vi "dlw_Message Log.vi"(6 "Worker Alias":string="Message Log", 7 "Caller in":refnum<class "Worker.lvclass">, 8 "error in":errorcluster, 9 "Initialization Data":T1, 11 "Message Log in":refnum<class "Message Log.lvclass">) -> (0 "error out":errorcluster, 3 "Message Log out":refnum<class "Message Log.lvclass">, 5 "dup Caller out":refnum<class "Worker.lvclass">)   [LabVIEW 2017, in "Message Log.lvclass"]
doc: "This VI dynamically loads the Worker that owns this VI as a subWorker into <b>Caller</b>, and returns the Worker's object containing the Worker's Public Properties. Initialization data that is to be received by this Worker's <Initialize> MHL case can be wired to <b>Initialization Data</b>. The dynamically loaded Worker requires an alias ( <b>Worker Alias</b> ) which must be unique to the Worker it is called from. If a currently loaded subWorker exists with the same Alias, an error will be returned.\n\n<b>Note:</b> This VI can only be called from <b>within</b> another Worker. To call this Worker from an external LabVIEW application, load this Worker with an Asynchronous Launcher VI.\n---"
uses:
  Message Log.lvclass
  C:/Program Files (x86)/National Instruments/LabVIEW 2017/vi.lib/addons/_Workers/Library/Classes/Worker/Worker.lvclass
  <vilib>/addons/_Workers/Library/Classes/Worker/Worker.lvclass
  Initialization Data.ctl
  Response Cases.ctl
  <vilib>/addons/_Workers/Library/Case Label.ctl
  Common VIs/Message Log ID.ctl
  Config Data.ctl
  <vilib>/Utility/miscctls.llb/LVRectTypeDef.ctl
  <vilib>/addons/_Workers/Library/Workers.lvlib
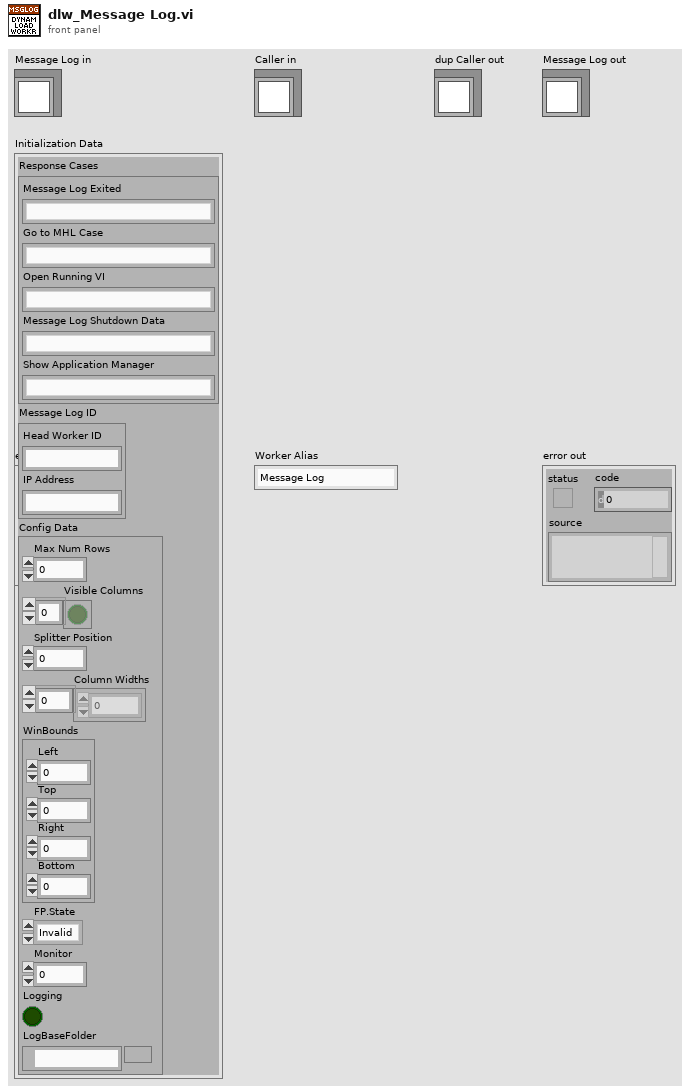
[diagram p1: front panel]
types:
  T1 = typedef "Message Log.lvclass/Initialization Data.ctl" = cluster{"Response Cases":T2, "Message Log ID":T4, "Config Data":T5}
  T2 = typedef "Message Log.lvclass/Response Cases.ctl" = cluster{"Message Log Exited":T3, "Go to MHL Case":T3, "Open Running VI":T3, "Message Log Shutdown Data":T3, "Show Application Manager":T3}
  T3 = typedef "Workers.lvlib/Case Label.ctl" = string
  T4 = typedef "Message Log ID.ctl" = cluster{"Head Worker ID":string, "IP Address":string}
  T5 = typedef "Message Log.lvclass/Config Data.ctl" = cluster{"Max Num Rows":i32, "Visible Columns":bool[], "Splitter Position":i32, "Column Widths":u32[], "WinBounds":T6, "FP.State":enum32{"Invalid", "Standard", "Closed", "Hidden", "Minimized", "Maximized"}, "Monitor":u16, "Logging":bool, "LogBaseFolder":path}
  T6 = typedef "LVRectTypeDef.ctl" = cluster{"Left":i16, "Top":i16, "Right":i16, "Bottom":i16}
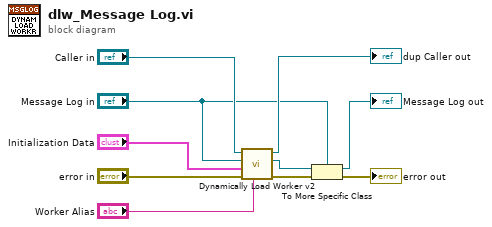
[diagram p0: block diagram]
diagram:
  n1 = call <vilib>:"Dynamically Load Worker v2.vi"("Worker Alias"="Worker Alias", "error in"="error in", "Initialization Data"="Initialization Data", "Worker to Dynamically Load"="Message Log in", "Worker"="Caller in") -> ("error out"=w9:errorcluster, "Dynamically Loaded Worker out"=w3:refnum<class "Worker.lvclass">, "dup Worker out"=→"dup Caller out":refnum<class "Worker.lvclass">)  [unwired: 4 in]
  n2 = To More Specific Class(target class="Message Log in", reference=w3, error in=w9) -> (specific class reference=→"Message Log out":refnum<class "Message Log.lvclass">, error out=→"error out":errorcluster)
